vi "cm_Overload Channels Popup.vi"() -> ()   [LabVIEW 2009, in "Channel Monitor.xctl"]
uses:
  Channel Monitor.xctl
  <vilib>/Utility/error.llb/DialogType.ctl
panel:
  in  "Threshold (% of Range)":dbl(slide) scale=0.0..100.0
  in  "Overloaded Channels":i32(listbox)
  out "error out":errorcluster
  in  "Close":bool
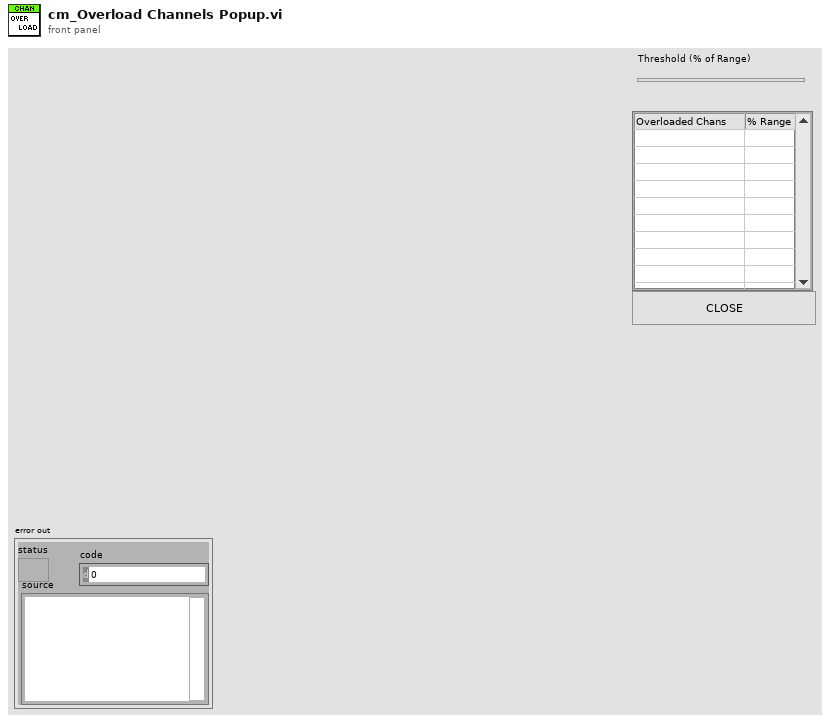
[diagram p1: front panel]
types:
  T1 = typedef "amc_Message Queue.ctl" = refnum<queue>
  T2 = cluster{"% of Range":dbl, "Index":i32, "Name":string}[]
  T3 = typedef "DialogType.ctl" = u16
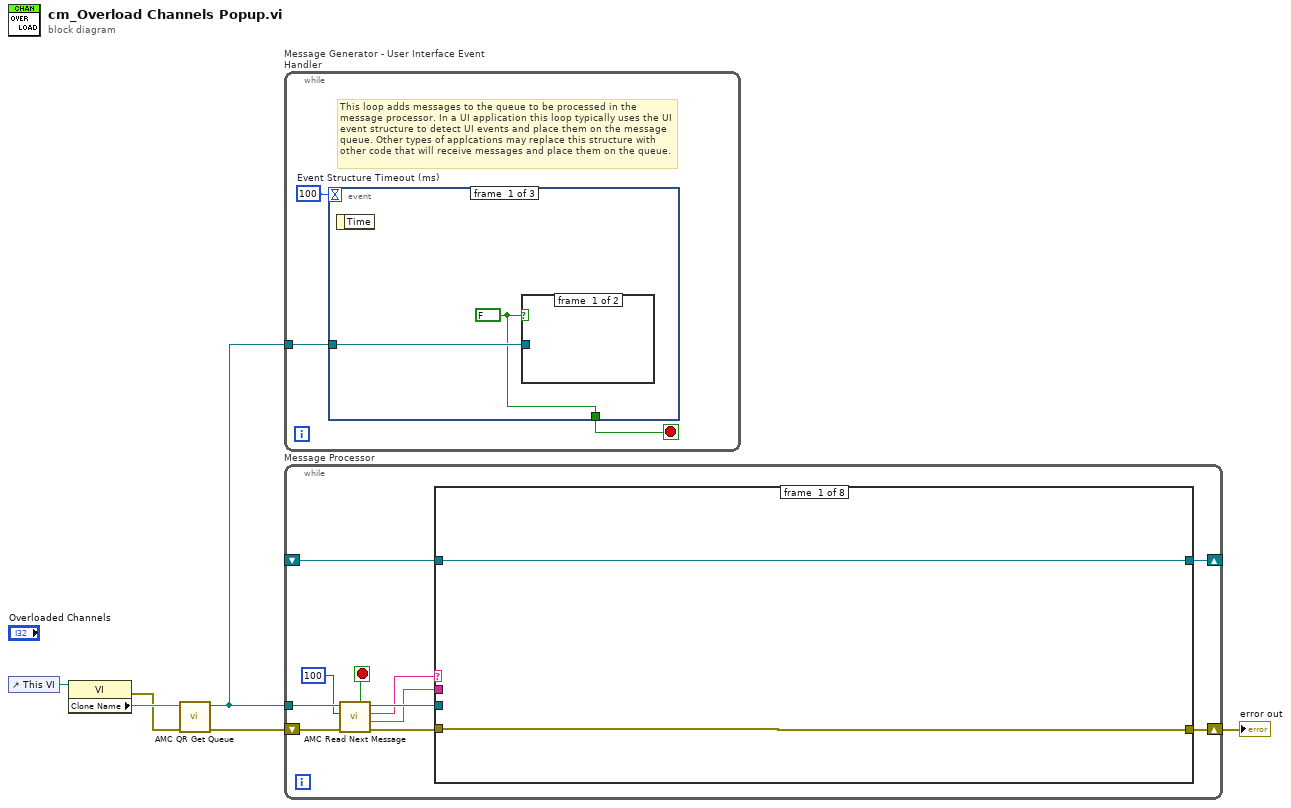
[diagram p0: block diagram]
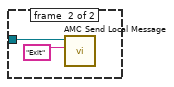
[diagram p2: hidden frame]
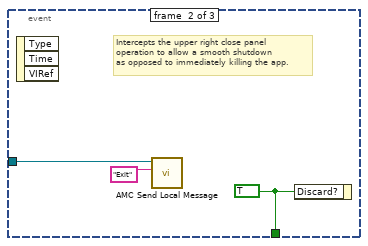
[diagram p3: hidden frame]
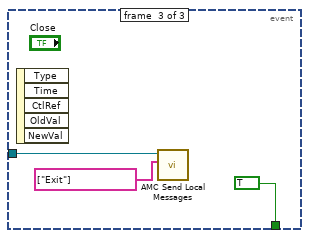
[diagram p4: hidden frame]
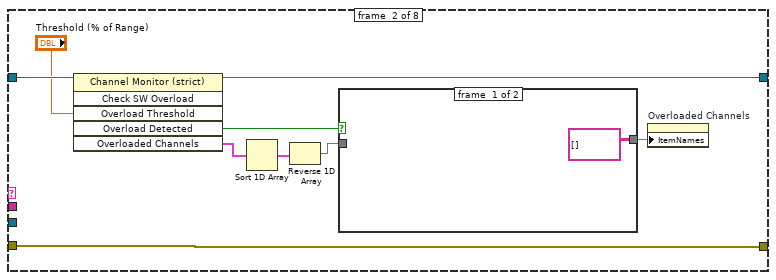
[diagram p5: hidden frame]
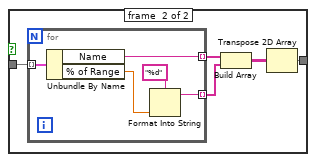
[diagram p6: hidden frame]
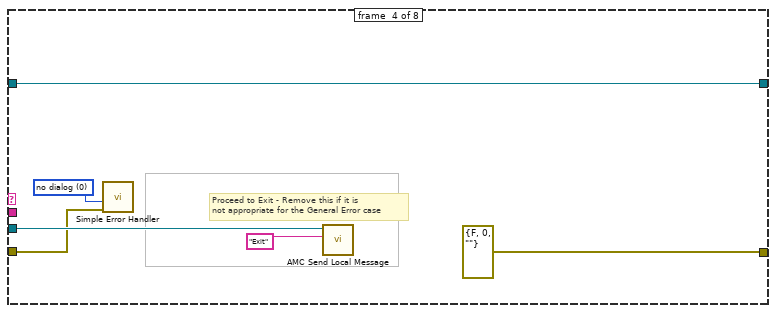
[diagram p8: hidden frame]
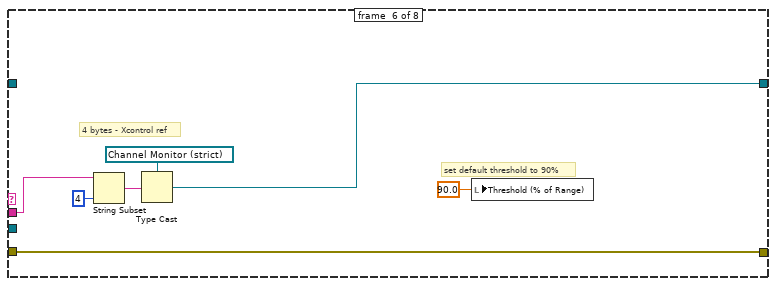
[diagram p10: hidden frame]
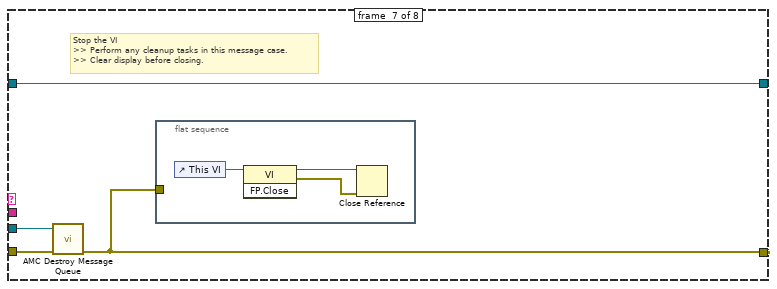
[diagram p11: hidden frame]
diagram:
  n1 = control-ref of="This VI"() -> (w4:refnum<vi>)
  n2 = property class="VI"(reference=w4) -> (error out=w1:errorcluster, "Clone Name"=w5:string)  [unwired: 1 in, 1 out]
  n3 = call <userlib>:"AMC QR Get Queue .vi"("error in (no error)"=w1, "Name"=w5) -> ("error out"=w2:errorcluster, "Queue Out"=w6:T1)  [unwired: 8 in]
  n4 = while "Message Generator - User Interface Event Handler" {
    tunnel: w6 -> [w7]
    stop <- w8 stop-if-true
    w9 = 100  # Event Structure Timeout (ms)
    # "This loop adds messages to the queue to be processed in the message processor. In a UI application this loop typically uses the UI event structure to detect UI events and place them on the message queue. Other types of applcations may replace this structure with other code that will receive messages and place them on the queue."
    n5 = event shown="[2] \"Close\": Value Change" {
      selector: _ -> [_ _ _]
      dyn-events: _ -> [_ _ _]
      timeout: w9 -> [_ _ _]
      tunnel: [w10 w16 TRUE ("Discard?")] -> w8
      tunnel: w7 -> [w11 w15 w18]
      event #0 {
        w10 = FALSE
        n6 = event-data() -> ()  [unwired: 2 out]
        n7 = case shown="True" w10 {
          tunnel: w11 -> [_ w12]
          frame #0 {
          }
          frame #1 {
            n8 = call <userlib>:"AMC Send Local Message.vi"("Message Name"="Exit", "Message Queue in"=w12) -> ()  [unwired: 4 in, 6 out]
          }
        }
      }
      event #1 {
        w16 = TRUE ("Discard?")
        # "Intercepts the upper right close panel\noperation to allow a smooth shutdown\nas opposed to immediately killing the app."
        n9 = event-data() -> ()  [unwired: 4 out]
        n10 = call <userlib>:"AMC Send Local Message.vi"("Message Name"="Exit", "Message Queue in"=w15) -> ()  [unwired: 4 in, 6 out]
        n11 = event-data("Discard?"=w16) -> ()  [unwired: 1 in, 1 out]
      }
      event #2 {
        n12 = event-data() -> ()  [unwired: 6 out]
        n13 = call <userlib>:"AMC Send Local Messages.vi"("Message Names"=string[] ["Exit"], "Message Queue in"=w18) -> ()  [unwired: 8 in, 2 out]
      }
    }
  }
  n14 = while "Message Processor" {
    shift-left: w2 -> [w29]
    shift-right: [w30] -> w3
    tunnel: w6 -> [w26]
    shift-right: [w21] -> _
    shift-left: _ -> [w20]
    stop <- w25 stop-if-true
    n15 = call <userlib>:"AMC Read Next Message.vi"("error in (no error)"=w29, "timeout (1ms)"=100, "Message Queue in"=w26) -> ("error out"=w28:errorcluster, "Message Value"=w23:string, "Message Name"=w24:string, "Message Queue out"=w27:T1, "Exit Process"=w25:bool)  [unwired: 1 in, 3 out]
    n16 = case shown="\"\", \"Idle\"" w24 {
      tunnel: w23 -> [_ _ _ _ _ w66 _ _]
      tunnel: w28 -> [w32 w41 w54 w57 w62 w65 w72 w78]
      tunnel: [w32 w41 w54 errorcluster {"status"=FALSE, "code"=0, "source"=""} ("error out") w62 w65 w71 w78] -> w30
      tunnel: w27 -> [_ _ _ w59 _ _ w73 _]
      tunnel: [w31 w39 w53 w55 w61 w64 w70 w77] -> w21
      tunnel: w20 -> [w31 w40 w53 w55 w61 _ w70 w77]
      frame #0 {
        # "Dummy case to add a seperator in the Case Structure menu"
      }
      frame #1 {
        n17 = invoke class="Channel Monitor (strict)" method="Check SW Overload"(reference=w40, "Overload Threshold"="Threshold (% of Range)") -> (reference out=w39:refnum<vi>, "Overload Detected"=w38:bool, "Overloaded Channels"=w35:T2)  [unwired: 4 in, 3 out]
        n18 = Sort 1D Array(array=w35) -> (sorted array=w33:T2)
        n19 = Reverse 1D Array(array=w33) -> (reversed array=w34:T2)
        n20 = case shown="True" w38 {
          tunnel: w34 -> [_ w47]
          tunnel: [string[][] [] w44] -> w37
          frame #0 {
          }
          frame #1 {
            n21 = for {
              tunnel: w47 -> [w49] mode=indexing
              tunnel: [w51] -> w46 mode=indexing
              tunnel: [w50] -> w43 mode=indexing
              n22 = Unbundle By Name(w49) -> ("Name"=w50:string, "% of Range"=w48:dbl)
              n23 = Format Into String(format string="%d", w48) -> (resulting string=w51:string)  [unwired: 2 in, 1 out]
            }
            n24 = Build Array(w43, w46) -> (w45:string[][])
            n25 = Transpose 2D Array(2D array=w45) -> (transposed array=w44:string[][])
          }
        }
        n26 = property on="Overloaded Channels" class="MCListbox (strict)"("ItemNames"=w37) -> ()  [unwired: 2 in, 2 out]
      }
      frame #2 {
        # "Call this case if a message is received that is not handled \nby any other case. Typically this is a programming error\nas a result of a typo or unhandled message/missing message handler."
      }
      frame #3 {
        w58 = T3 0 items=["no dialog", "OK message", "continue or stop message", "OK message + warnings", "continue/stop + warnings"] ("type of dialog (OK msg:1)")
        # "Proceed to Exit - Remove this if it is\nnot appropriate for the General Error case"
        # "General Error Case - this case is called if an error is passed using the error cluster below. Typically most new errors should be handed in each individual case and not passed in the rror cluster. If necessary a custom error handler case should be added and called from other cases."
        n27 = call <vilib>:"Simple Error Handler.vi"("type of dialog (OK msg:1)"=w58, "error in (no error)"=w57) -> ()  [unwired: 8 out]
        n28 = call <userlib>:"AMC Send Local Message.vi"("Message Name"="Exit", "Message Queue in"=w59) -> ()  [unwired: 4 in, 6 out]
      }
      frame #4 {
        # "Dummy case to add a seperator in the Case Structure menu"
      }
      frame #5 {
        # "set default threshold to 90%"
        # "4 bytes - Xcontrol ref"
        # "Initialize the state variables and user interface"
        n29 = String Subset(string=w66, length (rest)=4 ("length (rest)")) -> (substring=w68:string)  [unwired: 1 in]
        n30 = Type Cast(type=refnum<vi> refnum ("Channel Monitor"), x=w68) -> (*(type *) &x=w64:refnum<vi>)
        n31 = local write "Threshold (% of Range)"(90.0 ("Threshold (% of Range)")) -> ()
      }
      frame #6 {
        # "Stop the VI\n>> Perform any cleanup tasks in this message case.\n>> Clear display before closing."
        n32 = call <userlib>:"AMC Destroy Message Queue.vi"("error in (no error)"=w72, "Message Queue in"=w73) -> ("error out"=w71:errorcluster)  [unwired: 9 out]
        n33 = flat-sequence {
          tunnel: w71 -> [_]
          frame #0 {
            n34 = control-ref of="This VI"() -> (w74:refnum<vi>)
            n35 = invoke class="VI" method="FP.Close"(reference=w74) -> (reference out=w76:refnum<vi>, error out=w75:errorcluster)  [unwired: 2 in, 1 out]
            n36 = Close Reference(reference=w76, error in (no error)=w75) -> ()  [unwired: 1 out]
          }
        }
      }
      frame #7 {
        # "Dummy case to add a seperator in the Case Structure menu"
      }
    }
  }
  "error out" <- w3
